vi "CT-Test (basic).vi"() -> ()   [LabVIEW 2015]
uses:
  Utility VIs/Math VIs/FFT x(t) to dB,Degrees (1D).vi
  HCT-Phase Enum.ctl
  HCT-Params.ctl
  HCT-Runtime Data.ctl
panel:
  in  "F0 (Hz)":dbl=400.0
  out "HCT Runtime":T1
  out "Time":cluster{"Array":dbl[], "Array":dbl[]}(graph)
  out "Freq":cluster{"Array":dbl[], "Array":dbl[]}(graph)
  in  "Frame size (ms)":dbl=100.0
  in  "Fs (Hz)":dbl=50000.0
  in  "HCT Params":T2={"F0 (Hz)"=500.0, "Band"={"Flow (Hz)"=800.0, "Fhigh (Hz)"=8000.0}, "Phase"=enum."Cosine", "Min F0 (Hz)"=400.0, "Max F0 (Hz)"=800.0}
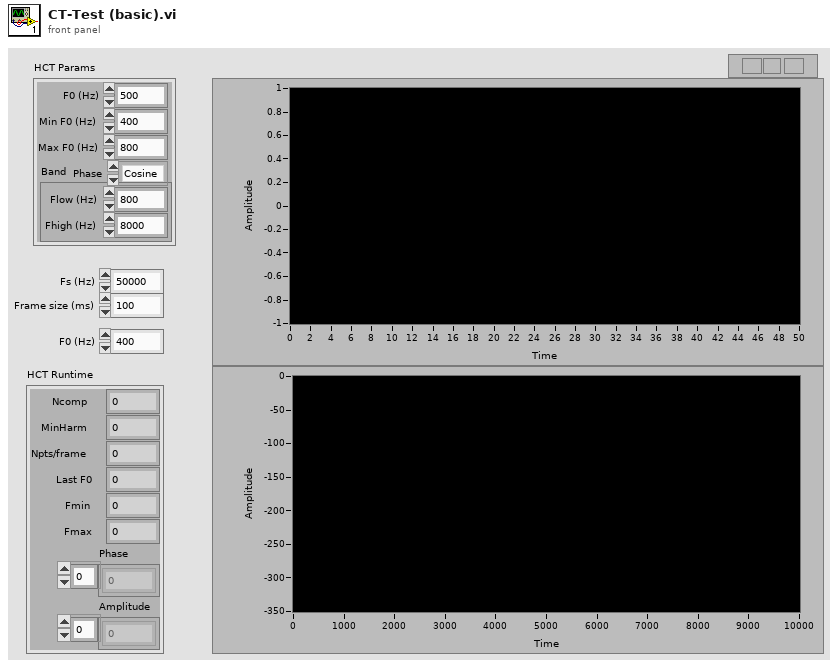
[diagram p1: front panel]
types:
  T1 = typedef "HCT-Runtime Data.ctl" = cluster{"Ncomp":i32, "MinHarm":i32, "Phase":dbl[], "Amplitude":dbl[], "Npts/frame":i32, "Last F0":dbl, "Fmin":dbl, "Fmax":dbl}
  T2 = typedef "HCT-Params.ctl" = cluster{"F0 (Hz)":dbl, "Band":cluster{"Flow (Hz)":dbl, "Fhigh (Hz)":dbl}, "Phase":T3, "Min F0 (Hz)":dbl, "Max F0 (Hz)":dbl}
  T3 = typedef "HCT-Phase Enum.ctl" = enum16{"Cosine", "Random", "Alternating"}
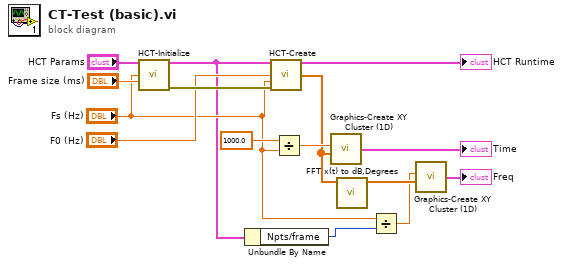
[diagram p0: block diagram]
diagram:
  n1 = call "HCT-Initialize.vi"("HCT Params"="HCT Params", "Fs (Hz)"="Fs (Hz)", "Frame size (ms)"="Frame size (ms)") -> ("HCT Runtime"=w5:T1, "error out"=w12:errorcluster)  [unwired: 11 in]
  n2 = Unbundle By Name(w5) -> ("Npts/frame"=w4:i32)
  n3 = call "HCT-Create.vi"("HCT Runtime in"=w5, "F0 (Hz)"="F0 (Hz)", "Fs (Hz)"="Fs (Hz)", "error in (no error)"=w12) -> ("HCT Runtime out"=→"HCT Runtime":T1, "HCT"=w7:dbl[])  [unwired: 9 in, 1 out]
  n4 = Divide(x=1000.0, y="Fs (Hz)") -> (x/y=w9:dbl)
  n5 = call "Graphics-Create XY Cluster (1D).vi"("Array"=w7, "dx"=w9) -> ("XY cluster"=→"Time":cluster{"Array":dbl[], "Array":dbl[]})  [unwired: 2 in]
  n6 = call-poly "FFT x(t) to dB,Degrees.vi"("X"=w7) -> ("+Freq. Mag of FFT (dB rms)"=w3:dbl[])  [unwired: 8 in, 2 out]
  n7 = Divide(x="Fs (Hz)", y=w4) -> (x/y=w2:dbl)
  n8 = call "Graphics-Create XY Cluster (1D).vi"("Array"=w3, "dx"=w2) -> ("XY cluster"=→"Freq":cluster{"Array":dbl[], "Array":dbl[]})  [unwired: 2 in]
